vi "Create Frame Pattern Script.vi"(8 "error in (no error)":errorcluster, 9 "ChipID":u8, 10 "Frame_Data":T1={"Pattern_Name"="", "Operation Mode"=enum."Normal", "BurstLength"=enum."0", "FSN"=0, "Start_Addr"=0, "Data"=[], "R/W?"=enum."Read", "Opcode"=[], "ChipID"=1, "num of wait cycle of read"=0} {"Data" format="%x"; "Start_Addr" format="%x"}, 11 "BML_Frame_Write in":refnum<class "BML_Frame_Write.lvclass">) -> (0 "error out":errorcluster, 3 "BML_Frame_Write out":refnum<class "BML_Frame_Write.lvclass">)   [LabVIEW 2018, in "BML_Frame_Write.lvclass"]
uses:
  BML_Frame_Write.lvclass
  C:/P4 Workspace/PC Client/Solutions/5g_eap/HiSi/trunk/1.0/BML_Pattern_Gen_Refactor/Classes/BML_Frame_Root/BML_Frame_Root.lvclass
  Config_Read/Frame_Data.ctl
  Config_Read/OperationMode.ctl
  Config_Read/BurstLength.ctl
  Config_Read/RW_Option.ctl
  BML_Frame_Root/Special Frame.ctl
  BML_Frame_Write.lvclass/BML_Frame_Write.ctl
  BML_Frame_Root/BML_Frame_Root.lvclass/BML_Frame_Root.ctl
  BML_Frame_Cmd/BML_Frame_Command.lvclass
  BML_Frame_Addr/BML_Frame_Addr.lvclass
  BML_Frame_Data/BML_Frame_Data.lvclass
  BML_Frame_Root/BML_Frame_Root.lvclass
  Config_Read/Config_Read_BML.lvclass
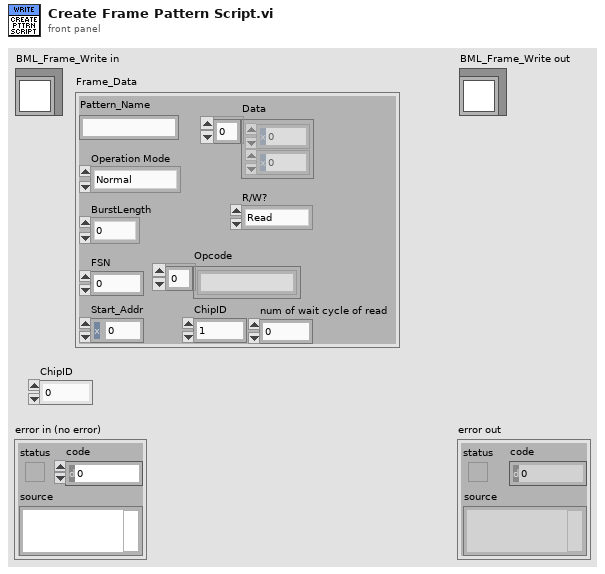
[diagram p1: front panel]
types:
  T1 = typedef "Config_Read_BML.lvclass/Frame_Data.ctl" = cluster{"Pattern_Name":string, "Operation Mode":T2, "BurstLength":T3, "FSN":u8, "Start_Addr":u16, "Data":u8[], "R/W?":T4, "Opcode":string[], "ChipID":u8, "num of wait cycle of read":i8}
  T2 = typedef "Config_Read_BML.lvclass/OperationMode.ctl" = enum8{"Normal", "ImmeEffect", "InitSlaveID", "LoadData"}
  T3 = typedef "Config_Read_BML.lvclass/BurstLength.ctl" = enum8{"0", "2", "3", "4", "5", "8", "16", "32"}
  T4 = typedef "Config_Read_BML.lvclass/RW_Option.ctl" = enum16{"Read", "Write", "R/W"}
  T5 = typedef "BML_Frame_Root.lvclass/Special Frame.ctl" = enum16{"Sync Header", "Protocol Header", "SW Trig", "SetID State", "Out SetID State", "SW Reset", "Wait", "SPI 4W FRM Start", "SPI 4W Wait", "SPI 4W FRM End", "SPI 4W Write Cmd", "SPI RD Collect Cmd", "SPI RD Value Cmd", "SPI 3W FRM Start", "SPI 3W Write Cmd", "SPI 3W FRM End", "SPI 3W Wait", "SPI 3W RD Cmd"}
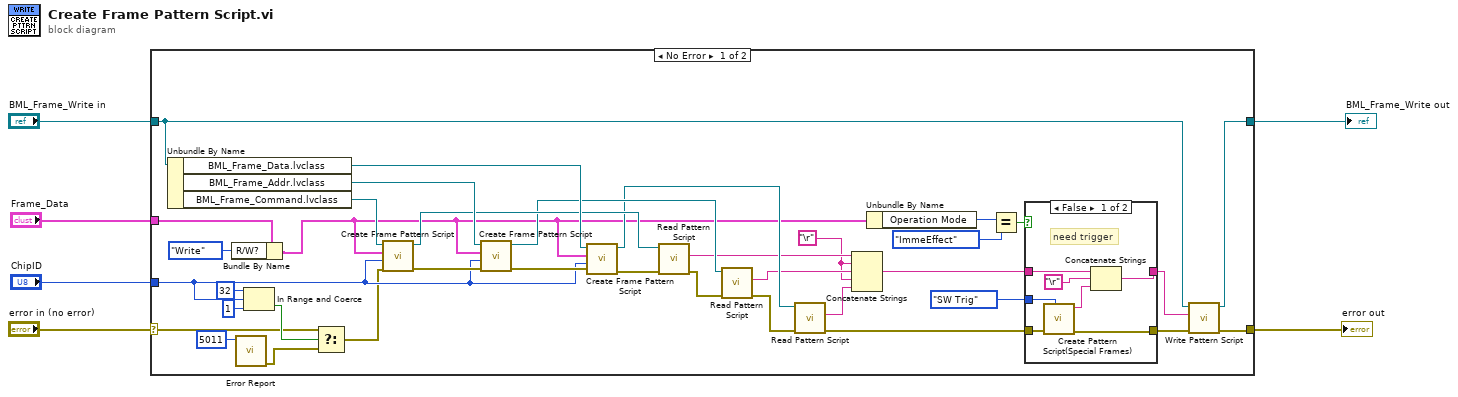
[diagram p0: block diagram]
diagram:
  n1 = case shown="No Error" "error in (no error)" {
    selector: "error in (no error)" -> [w10 w54]
    tunnel: [w18 w54] -> w5
    tunnel: "BML_Frame_Write in" -> [w20 w53]
    tunnel: [w19 w53] -> w3
    tunnel: "Frame_Data" -> [w17 _]
    tunnel: "ChipID" -> [w11 _]
    frame No Error {
      w30 = "\r"
      n2 = Unbundle By Name(w20) -> ("BML_Frame_Data.lvclass"=w39:refnum<class "BML_Frame_Data.lvclass">, "BML_Frame_Addr.lvclass"=w40:refnum<class "BML_Frame_Addr.lvclass">, "BML_Frame_Command.lvclass"=w41:refnum<class "BML_Frame_Command.lvclass">)
      n3 = Bundle By Name(cluster=w17, "R/W?"=RW_Option."Write") -> (w15:T1)
      n4 = call "Error Report.vi"("Error Code"=i16 5011) -> ("error out"=w9:errorcluster)  [unwired: 10 in]
      n5 = In Range and Coerce(upper limit=u8 32, x=w11, lower limit=u8 1) -> (In Range?=w13:bool)  [unwired: 1 out]
      n6 = Select(t=w10, s=w13, f=w9) -> (s? t:f=w8:errorcluster)
      n7 = call-dynamic "Create Frame Pattern Script.vi"("error in (no error)"=w8, "ChipID"=w11, "Frame_Data"=w15, "BML_Frame_Command in"=w41) -> ("error out"=w43:errorcluster, "BML_Frame_Command out"=w37:refnum<class "BML_Frame_Command.lvclass">)  [unwired: 6 in]
      n8 = call-dynamic "Create Frame Pattern Script.vi"("error in (no error)"=w43, "ChipID"=w11, "Frame_Data"=w15, "BML_Frame_Addr in"=w40) -> ("error out"=w42:errorcluster, "BML_Frame_Addr out"=w35:refnum<class "BML_Frame_Addr.lvclass">)  [unwired: 6 in]
      n9 = call-dynamic "Create Frame Pattern Script.vi"("error in (no error)"=w42, "ChipID"=w11, "Frame_Data"=w15, "BML_Frame_Data in"=w39) -> ("error out"=w38:errorcluster, "BML_Frame_Data out"=w34:refnum<class "BML_Frame_Data.lvclass">)  [unwired: 6 in]
      n10 = call "Read Pattern Script.vi"("error in (no error)"=w38, "BML_Frame_Root in"=w37) -> ("error out"=w36:errorcluster, "Pattern Script"=w32:string)  [unwired: 7 in, 1 out]
      n11 = call "Read Pattern Script.vi"("error in (no error)"=w36, "BML_Frame_Root in"=w35) -> ("error out"=w33:errorcluster, "Pattern Script"=w31:string)  [unwired: 7 in, 1 out]
      n12 = call "Read Pattern Script.vi"("error in (no error)"=w33, "BML_Frame_Root in"=w34) -> ("error out"=w24:errorcluster, "Pattern Script"=w29:string)  [unwired: 7 in, 1 out]
      n13 = Concatenate Strings(w32, w30, w31, w30, w29) -> (w25:string)
      n14 = Unbundle By Name(w15) -> ("Operation Mode"=w28:T2)
      n15 = Equal?(x=w28, y=OperationMode."ImmeEffect") -> (x = y?=w26:bool)
      n16 = case shown="False" w26 {
        tunnel: w25 -> [w47 w52]
        tunnel: w24 -> [w50 w51]
        tunnel: [w48 w52] -> w21
        tunnel: [w46 w51] -> w22
        tunnel: Special_Frame."SW Trig" ("Special Frame Type") -> [w49 _]
        frame False {
          # "need trigger"
          n17 = call "Create Pattern Script(Special Frames).vi"("Special Frame Type"=w49, "error in (no error)"=w50) -> ("error out"=w46:errorcluster, "string out"=w45:string)  [unwired: 8 in]
          n18 = Concatenate Strings(w47, "\r", w45) -> (w48:string)
        }
        frame True {
        }
      }
      n19 = call "Write Pattern Script.vi"("error in (no error)"=w22, "Pattern Script"=w21, "BML_Frame_Root in"=w20) -> ("error out"=w18:errorcluster, "BML_Frame_Root out"=w19:refnum<class "BML_Frame_Write.lvclass">)  [unwired: 7 in]
    }
    frame Error {
    }
  }
  "error out" <- w5
  "BML_Frame_Write out" <- w3
